vi "DetectPressureAnomalies.vi"(3 "Pressure Loss Threshold (psi/min)":dbl=-5.0, 4 "Compressor Running":bool, 5 "Pressure (psi)":dbl(slide) scale=0.0..120.0) -> (0 "Pressure Change (psi/min)":dbl, 1 "Pressure Leak":bool, 2 "Pressure Vent":bool)   [LabVIEW 2020]
doc: "This VI can detect both rapid pressure venting events and slow pressure leak conditions."
uses:
  012c8d05-766e-4104-b1bd-0e91dd28699c.vi
  GlobalDriverStationData.vi
  <vilib>/Analysis/NI_AALPro.lvlib
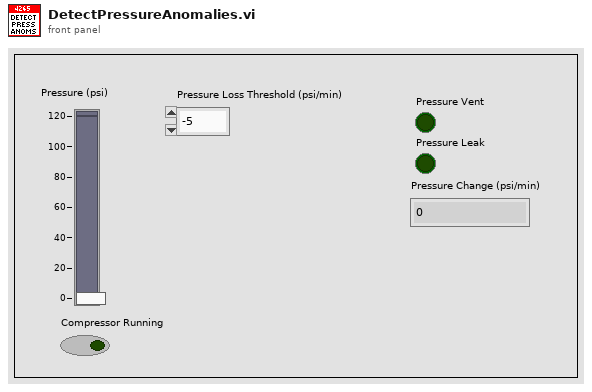
[diagram p1: front panel]
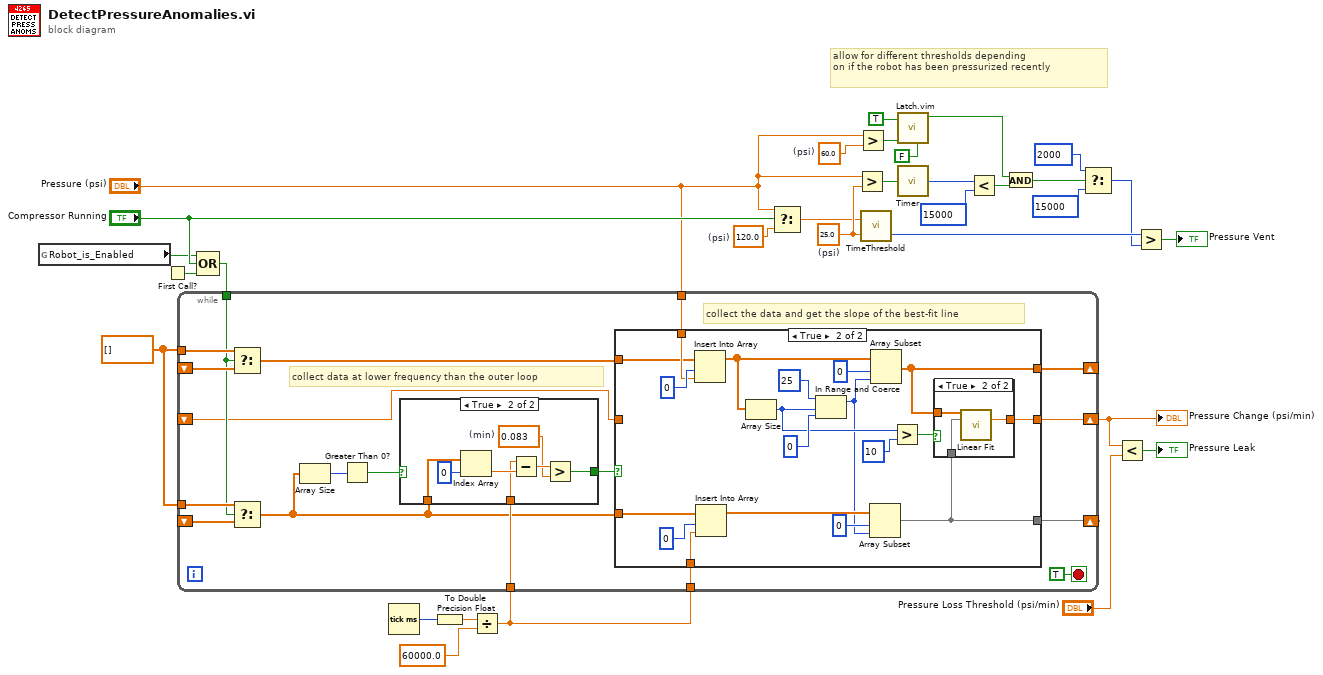
[diagram p0: block diagram]
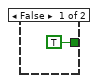
[diagram p2: hidden frame]
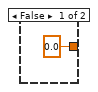
[diagram p4: hidden frame]
diagram:
  w4 = 60.0  # (psi)
  w22 = dbl[] [] ("array")
  w31 = 120.0  # (psi)
  w17 = 25.0  # (psi)
  # "allow for different thresholds depending\non if the robot has been pressurized recently"
  n1 = global read "GlobalDriverStationData.vi" "Robot_is_Enabled"() -> (w1:bool)
  n2 = First Call?() -> (First Call?: T/F=w28:bool)
  n3 = Compound Arithmetic op=OR(w1, "Compressor Running", w28) -> (w26:bool)
  n4 = Tick Count (ms)() -> (millisecond timer value=w25:u32)
  n5 = To Double Precision Float(number=w25) -> (double precision float=w24:dbl)
  n6 = Divide(x=w24, y=60000.0) -> (x/y=w18:dbl)
  n7 = while {
    tunnel: "Pressure (psi)" -> [w48]
    shift-right: [w45] -> _
    shift-left: _ -> [w47]
    tunnel: w22 -> [w46]
    tunnel: w26 -> [w40]
    tunnel: w18 -> [w42]
    tunnel: w22 -> [w41]
    shift-right: [w39] -> _
    shift-left: _ -> [w38]
    tunnel: w18 -> [w37]
    shift-right: [w44] -> w21
    shift-left: _ -> [w32]
    stop <- TRUE stop-if-true
    # "collect the data and get the slope of the best-fit line"
    # "collect data at lower frequency than the outer loop"
    n8 = Select(t=w46, s=w40, f=w47) -> (s? t:f=w43:dbl[])
    n9 = Select(t=w41, s=w40, f=w38) -> (s? t:f=w35:dbl[])
    n10 = Array Size(array=w35) -> (size(s)=w34:i32)
    n11 = Greater Than 0?(x=w34) -> (x > 0?=w33:bool)
    n12 = case shown="True" w33 {
      tunnel: w37 -> [_ w55]
      tunnel: [TRUE w52] -> w36
      tunnel: w35 -> [_ w51]
      frame False {
      }
      frame True {
        w53 = 0.083  # (min)
        n13 = Index Array(array=w51, index=0) -> (element=w56:dbl)
        n14 = Subtract(x=w55, y=w56) -> (x-y=w54:dbl)
        n15 = Greater?(x=w54, y=w53) -> (0:w52:bool)
      }
    }
    n16 = case shown="True" w36 {
      tunnel: w48 -> [_ w78]
      tunnel: [w60 w73] -> w45
      tunnel: [w58 w69] -> w44
      tunnel: w43 -> [w60 w67]
      tunnel: w42 -> [_ w66]
      tunnel: [w59 w62] -> w39
      tunnel: w35 -> [w59 w61]
      tunnel: w32 -> [w58 _]
      frame False {
      }
      frame True {
        n17 = Insert Into Array(array=w67, index=0, new element=w78) -> (w76:dbl[])
        n18 = Insert Into Array(array=w61, index=0, new element=w66) -> (w64:dbl[])
        n19 = Array Size(array=w76) -> (size(s)=w71:i32)
        n20 = In Range and Coerce(upper limit=25, x=w71, lower limit=0) -> (coerced(x)=w63:i32)  [unwired: 1 out]
        n21 = Array Subset(array=w64, index=0, length=w63) -> (w62:dbl[])
        n22 = Array Subset(array=w76, index=0, length=w63) -> (w73:dbl[])
        n23 = Greater?(x=w71, y=10) -> (0:w72:bool)
        n24 = case shown="True" w72 {
          tunnel: w73 -> [_ w83]
          tunnel: [0.0 ("slope") w82] -> w69
          tunnel: w62 -> [_ w81]
          frame False {
          }
          frame True {
            n25 = call <vilib>:"Linear Fit.vi"("Y"=w83, "X"=w81) -> ("slope"=w82:dbl)  [unwired: 9 in, 4 out]
          }
        }
      }
    }
  }
  "Pressure Change (psi/min)" <- w21
  n26 = Select(t="Pressure (psi)", s="Compressor Running", f=w31) -> (s? t:f=w5:dbl)
  n27 = Greater?(x="Pressure (psi)", y=w17) -> (0:w10:bool)
  n28 = Greater?(x="Pressure (psi)", y=w4) -> (0:w3:bool)
  n29 = call "TimeThreshold.vi"("Threshold"=w17, "Current Value"=w5) -> ("Time Below Threshold (ms)"=w30:u32)  [unwired: 1 out]
  n30 = call "Latch.vim"("Default Value"=FALSE, "Latch Signal"=w3, "Latch Value"=TRUE) -> ("Latched"=w7:bool)  [unwired: 8 in]
  n31 = call "Timer.vi"("Reset Timer"=w10) -> ("Time (ms)"=w16:u32)
  n32 = Less?(x=w16, y=u32 15000) -> (x < y?=w11:bool)
  n33 = And(x=w7, y=w11) -> (x .and. y?=w6:bool)
  n34 = Select(t=u32 2000 ("y"), s=w6, f=u32 15000) -> (s? t:f=w12:u32)
  n35 = Less?(x=w21, y="Pressure Loss Threshold (psi/min)") -> (x < y?=→"Pressure Leak":bool)
  n36 = Greater?(x=w30, y=w12) -> (0:→"Pressure Vent":bool)
